vi "read.vi"(8 "error in (no error)":errorcluster, 11 "UDP Tx in":refnum<class "UDP Tx.lvclass">) -> (0 "error out":errorcluster, 1 "Received Packet":bool=TRUE, 2 "Received data":string[](array[string]), 3 "UDP Tx out":refnum<class "UDP Tx.lvclass">)   [LabVIEW 2012, in "UDP Tx.lvclass"]
uses:
  UDP Tx.lvclass
  UDP Tx.lvclass/UDP Tx.ctl
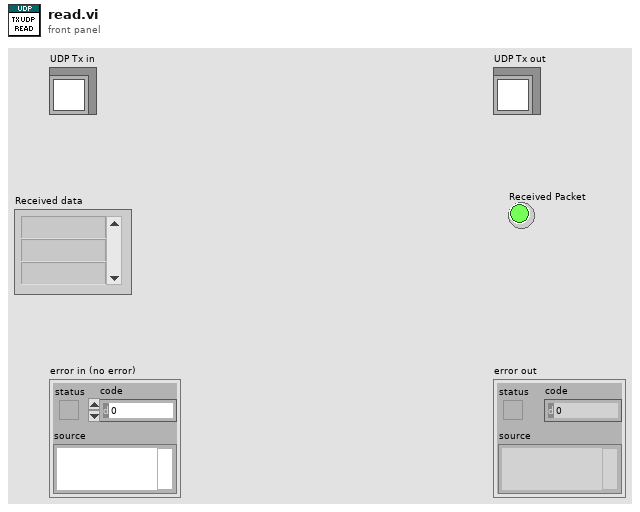
[diagram p1: front panel]
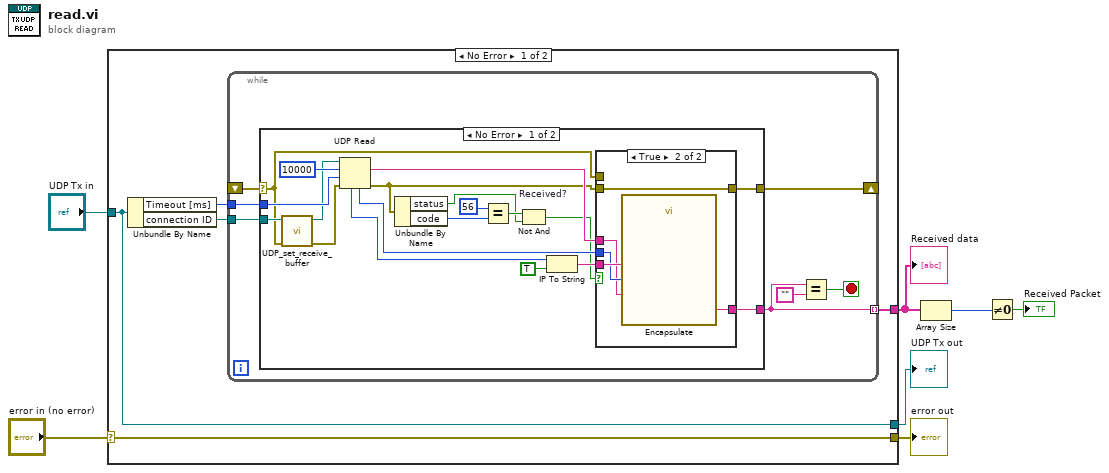
[diagram p0: block diagram]
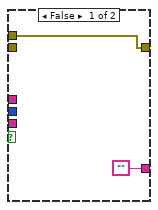
[diagram p2: hidden frame]
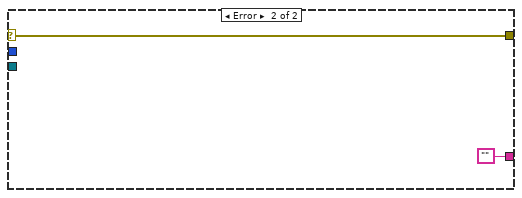
[diagram p3: hidden frame]
diagram:
  n1 = case shown="No Error" "error in (no error)" {
    selector: "error in (no error)" -> [w12 w49]
    tunnel: [w12 w49] -> w6
    tunnel: [w11 w48] -> w4
    tunnel: "UDP Tx in" -> [w11 w48]
    tunnel: [w8 _] -> w2
    frame No Error {
      n2 = Unbundle By Name(w11) -> ("Timeout [ms]"=w9:u16, "connection ID"=w10:refnum<k16>)
      n3 = while {
        tunnel: [w17] -> w8 mode=indexing
        shift-right: [w19] -> _
        shift-left: _ -> [w18]
        tunnel: w10 -> [w14]
        tunnel: w9 -> [w13]
        stop <- w15 stop-if-true
        n4 = case shown="No Error" w18 {
          selector: w18 -> [w22 w46]
          tunnel: [w36 ""] -> w17
          tunnel: [w27 w46] -> w19
          tunnel: w14 -> [w23 _]
          tunnel: w13 -> [w24 _]
          frame No Error {
            n5 = call "UDP_set_receive_buffer.vi"("error in (no error)"=w22, "connection ID"=w23) -> ("error out"=w20:errorcluster, "connection ID out"=w21:refnum<k16>)  [unwired: 7 in]
            n6 = UDP Read(connection ID=w21, max size (548)=10000, timeout ms (25000)=w24, 8:w20) -> (data out=w37:string, error out=w26:errorcluster, 4:w33:u16, 6:w25:u32)  [unwired: 1 out]
            n7 = Unbundle By Name(w26) -> ("status"=w28:bool, "code"=w31:i32)
            n8 = Equal?(x=56 ("y"), y=w31) -> (x = y?=w29:bool)
            n9 = Not And "Received?"(1:w28, 2:w29) -> (0:w30:bool)
            n10 = IP To String(1:TRUE ("dot notation? (F)"), 2:w25) -> (0:w34:string)
            n11 = case shown="True" w30 {
              tunnel: w37 -> [_ w42]
              tunnel: ["" w44] -> w36
              tunnel: w34 -> [_ w45]
              tunnel: w33 -> [_ w43]
              tunnel: [w39 w41] -> w27
              tunnel: w22 -> [w39 _]
              tunnel: w26 -> [_ w41]
              frame False {
              }
              frame True {
                n12 = call "Encapsulate"("src.ip"=w45, "src.port"=w43, "Packet Content"=w42) -> ("Result"=w44:string)  [unwired: 11 in, 1 out]
              }
            }
          }
          frame Error {
          }
        }
        n13 = Equal?(x=w17, y="") -> (x = y?=w15:bool)
      }
    }
    frame Error {
    }
  }
  "error out" <- w6
  "UDP Tx out" <- w4
  "Received data" <- w2
  n14 = Array Size(array=w2) -> (size(s)=w3:i32)
  n15 = Not Equal To 0?(x=w3) -> (x != 0?=→"Received Packet":bool)
